vi "LabViewTest_1.vi"() -> ()   [LabVIEW 2016]
panel:
  out "x+y":i32
  in  "Numeric":i32
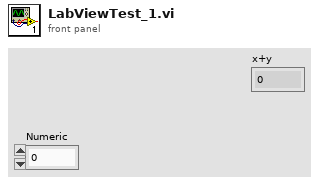
[diagram p1: front panel]
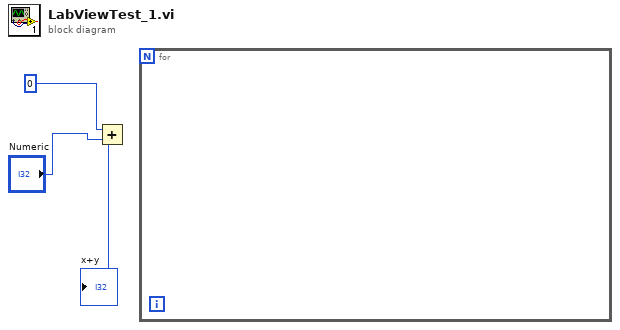
[diagram p0: block diagram]
diagram:
  n1 = Add(x=0, y="Numeric") -> (x+y=→"x+y":i32)
  n2 = for {
  }
